vi "Data File Processing UI Build Type and Data Messages.vi"(7 "type":T2, 13 "data":variant) -> (8 "msg out":T1[](array[typedef]))   [LabVIEW 2012]
uses:
  Data File Processing UI Message Type Define.ctl
  Data File Processing UI Message Define.ctl
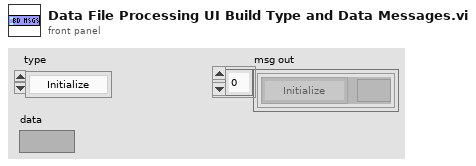
[diagram p1: front panel]
types:
  T1 = typedef "Data File Processing UI Message Define.ctl" = cluster{"data":variant, "type":T2}
  T2 = typedef "Data File Processing UI Message Type Define.ctl" = enum32{"Initialize", "SleepThread", "ErrorHandler", "NoEvent", "PreExit", "Exit", "----Action----", "OpenFile", "ReadAllCompute", "SaveFile", "RedrawGraph", "SelectChannel"}
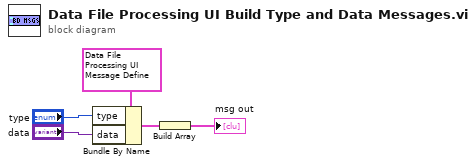
[diagram p0: block diagram]
diagram:
  n1 = Bundle By Name(cluster=T1 {"data"=variant, "type"=enum."Initialize"} ("MsgDef"), "type"="type", "data"="data") -> (w2:T1)
  n2 = Build Array(w2) -> (→"msg out":T1[])
